vi "Error_folder.vi"(1 "error in":errorcluster, 2 "File PNG":string[](array[string]), 3 "Folder Path":path) -> (0 "error out":errorcluster)   [LabVIEW 2025]
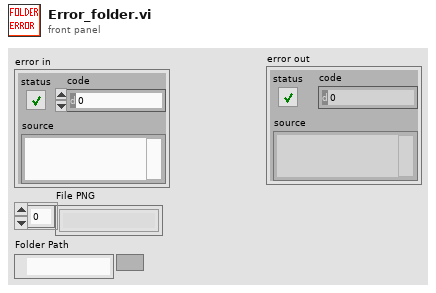
[diagram p1: front panel]
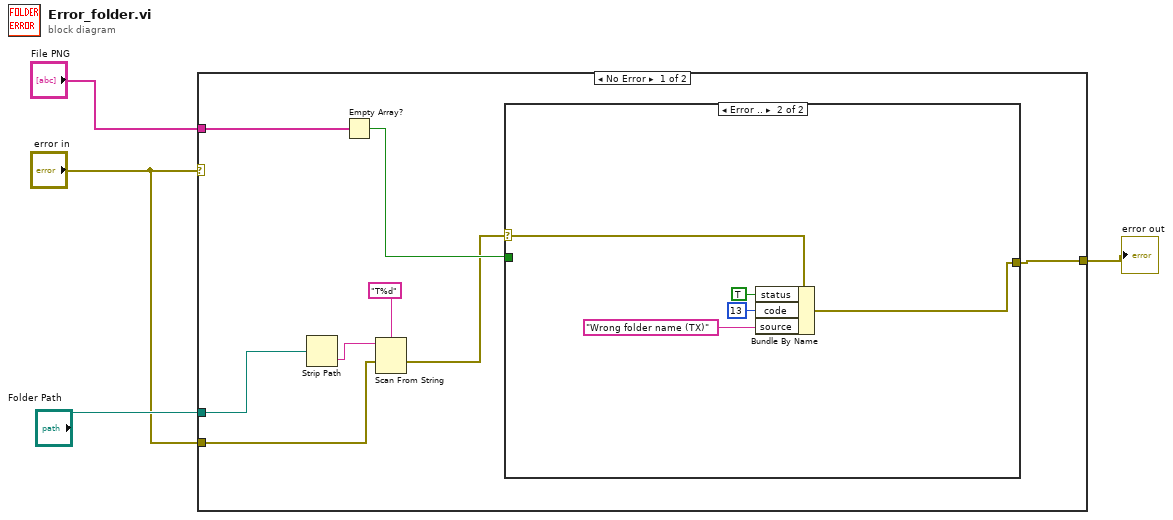
[diagram p0: block diagram]
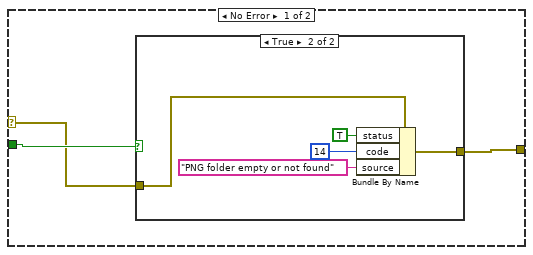
[diagram p2: hidden frame]
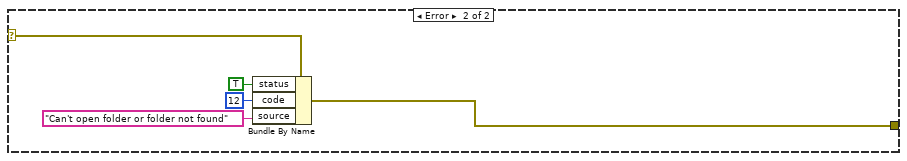
[diagram p4: hidden frame]
diagram:
  n1 = case shown="No Error" "error in" {
    selector: "error in" -> [_ w31]
    tunnel: "File PNG" -> [w10 _]
    tunnel: [w11 w30] -> w4
    tunnel: "Folder Path" -> [w7 _]
    tunnel: "error in" -> [w6 _]
    frame No Error {
      n2 = Strip Path(path=w7) -> (name=w9:string)  [unwired: 1 out]
      n3 = Empty Array?(array=w10) -> (empty?=w12:bool)
      n4 = Scan From String(format string="T%d", input string=w9, error in=w6) -> (error out=w5:errorcluster)  [unwired: 3 in, 2 out]
      n5 = case shown="Error .." w5 {
        selector: w5 -> [w13 w23]
        tunnel: w12 -> [w15 _]
        tunnel: [w14 w22] -> w11
        frame No Error {
          n6 = case shown="True" w15 {
            tunnel: w13 -> [w16 w18]
            tunnel: [w16 w17] -> w14
            frame False {
            }
            frame True {
              n7 = Bundle By Name(cluster=w18, "status"=TRUE, "code"=14, "source"="PNG folder empty or not found") -> (w17:errorcluster)
            }
          }
        }
        frame Error {
          n8 = Bundle By Name(cluster=w23, "status"=TRUE, "code"=13, "source"="Wrong folder name (TX)") -> (w22:errorcluster)
        }
      }
    }
    frame Error {
      n9 = Bundle By Name(cluster=w31, "status"=TRUE, "code"=12, "source"="Can't open folder or folder not found") -> (w30:errorcluster)
    }
  }
  "error out" <- w4
